vi "Outgoing Signals.vi"(8 "error in (no error)":errorcluster, 11 "Node Ptr":T4 format="%.0x") -> (0 "error out":errorcluster)   [LabVIEW 2009, in "NI-XNET Custom Device.lvlib"]
uses:
  NI-XNET Custom Device.lvlib
  <vilib>/NI VeriStand/Custom Device API/Custom Device Item Ref.ctl
  Add Selected.ctl
  Add All.ctl
  Browse for Channel.ctl
  <vilib>/xnet/xnet.llb/XNET String To IO Name (Frame).vi
  <vilib>/NI VeriStand/Custom Device API/Get Item Property (String).vi
  <vilib>/NI VeriStand/Custom Device API/Get Item Property (Boolean).vi
  <vilib>/NI VeriStand/Custom Device API/Custom Device Channel.ctl
  <vilib>/NI VeriStand/Custom Device API/Custom Device Channel Type.ctl
  <vilib>/NI VeriStand/Custom Device API/Set Item Property (Variant).vi
  <vilib>/NI VeriStand/Custom Device API/Set Item Property (Boolean).vi
  <vilib>/NI VeriStand/Custom Device API/Set Item Property (String).vi
  <vilib>/NI VeriStand/Custom Device API/Custom Device API.lvlib
  Program Files/National Instruments/LabVIEW 2009/resource/objmgr/xnet.rc
panel:
  in  "Enable Bool":bool
  in  "Header 6":cluster{"Section Name 2":string}={"Section Name 2"="Frame Timing"}
  out "Enable/Disable Channel":string
  in  "Add Enable":T1
  in  "Header 5":cluster{"Section Name":string}={"Section Name"="Signal Specifications"}
  in  "Header 4":cluster{"Section Name":string}={"Section Name"="Signal Values"}
  in  "Header 3":cluster{"Section Name":string}={"Section Name"="Signal Settings"}
  in  "Add All":T2
  in  "Add Signal":T3
  out "Unit":string
  out "Start Bit":u32
  out "Scaling Offset":dbl
  out "Scaling Factor":dbl
  out "Number of Bits":u32
  out "Minimum Value":dbl
  out "Maximum Value":dbl
  out "Default Value":dbl
  out "Data Type":u32(ring) items=["Signed", "Unsigned", "IEEE Float"]
  out "Comment":string
  out "Byte Order":u32(ring) items=["Little Endian", "Big Endian"]
  in  "Signal Selection":i32(listbox)
  in  "Header":cluster{"Section Name":string}={"Section Name"="Signal Selection"}
  in  "Delete":bool
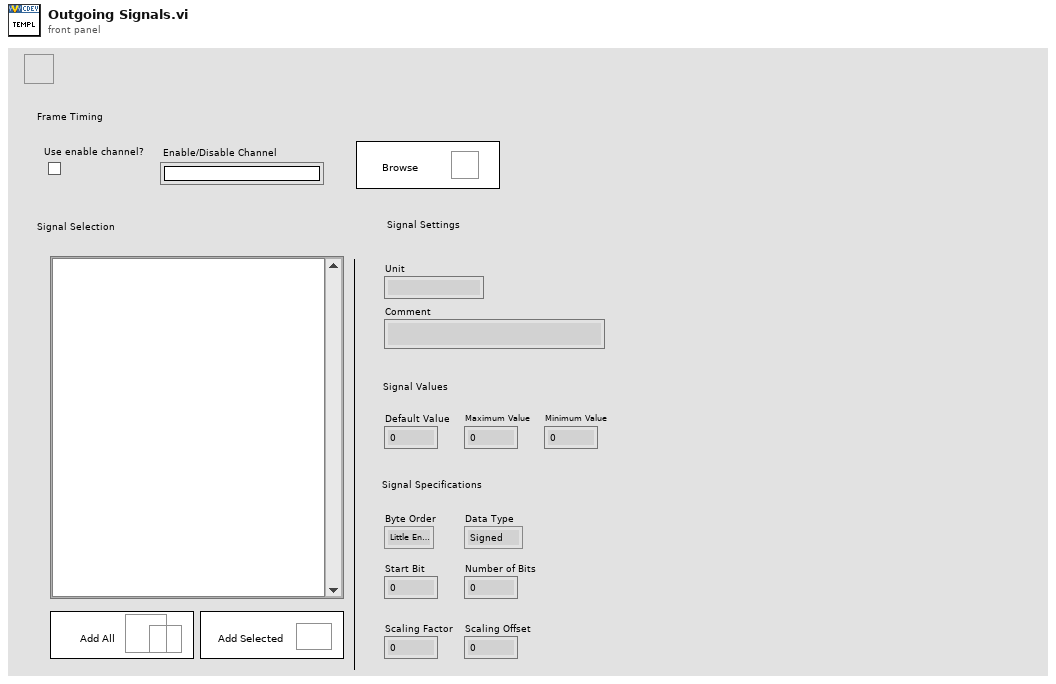
[diagram p1: front panel]
types:
  T1 = typedef "NI-XNET Custom Device.lvlib/Browse for Channel.ctl" = bool
  T2 = typedef "NI-XNET Custom Device.lvlib/Add All.ctl" = bool
  T3 = typedef "NI-XNET Custom Device.lvlib/Add Selected.ctl" = bool
  T4 = typedef "Custom Device API.lvlib/Custom Device Item Ref.ctl" = u64
  T5 = typedef "Custom Device API.lvlib/Custom Device Channel.ctl" = cluster{"Type":T6, "Units":string, "Default Value":dbl, "Faultable":bool, "Scalable":bool}
  T6 = typedef "Custom Device API.lvlib/Custom Device Channel Type.ctl" = enum16{"Input", "Output"}
  T7 = typedef "Custom Device API.lvlib/Custom Device Commands.ctl" = enum16{"Default", "Item renamed", "Shutdown"}
  T8 = typedef "Custom Device API.lvlib/Custom Device Item Info.ctl" = cluster{"Name":string, "Is Channel":bool, "GUID":string}
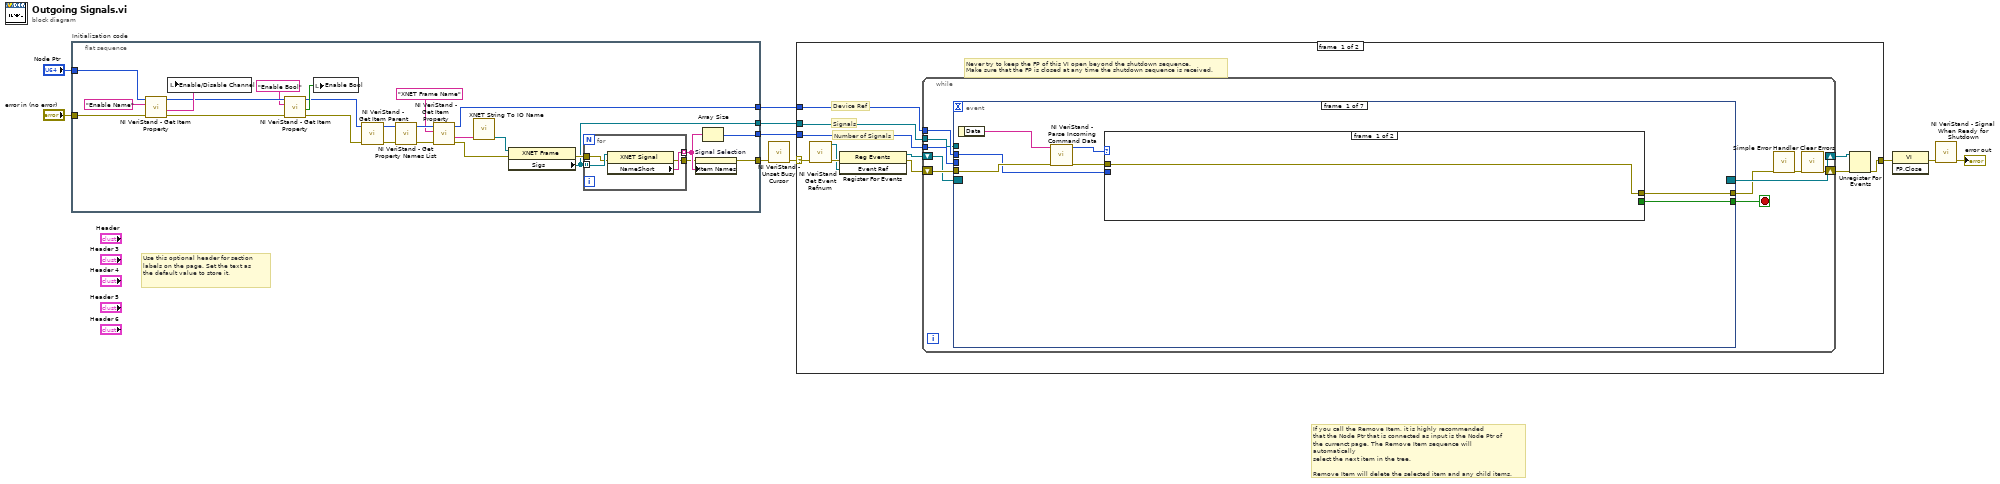
[diagram p0: block diagram]
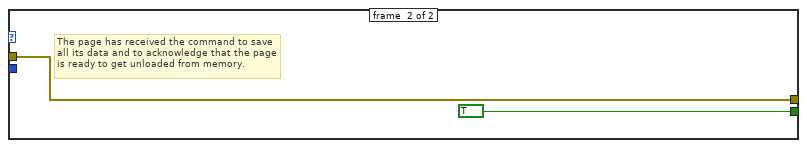
[diagram p2: hidden frame]
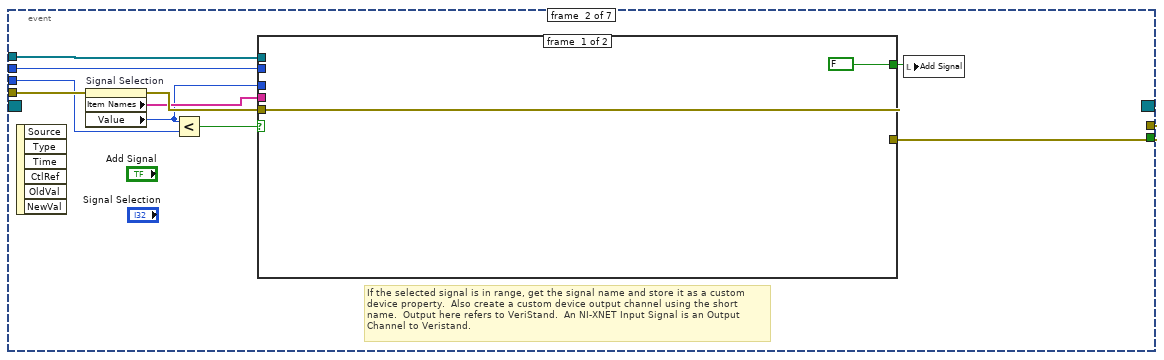
[diagram p3: hidden frame]
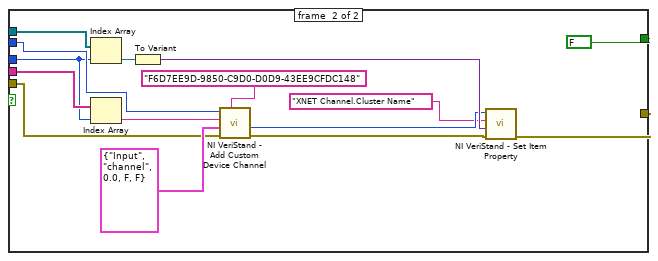
[diagram p4: hidden frame]
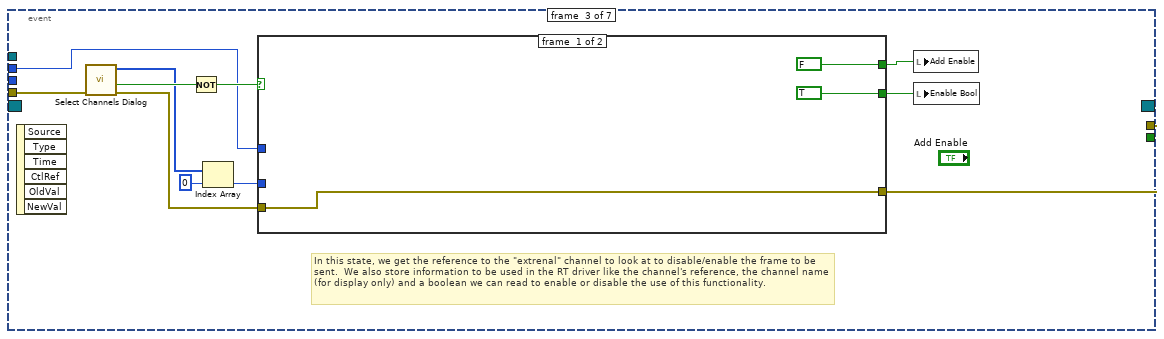
[diagram p5: hidden frame]
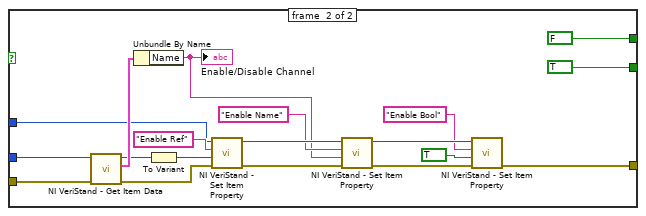
[diagram p6: hidden frame]
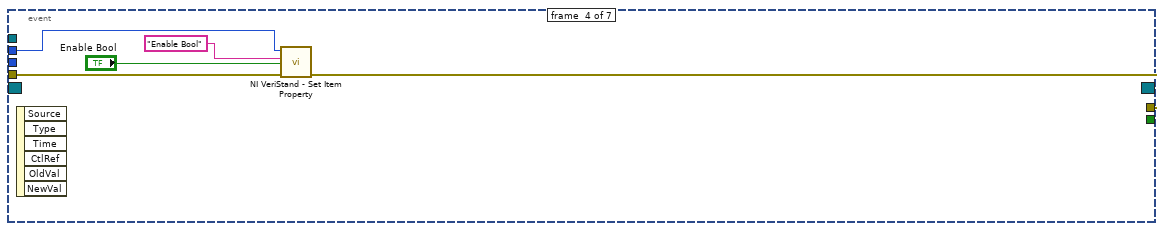
[diagram p7: hidden frame]
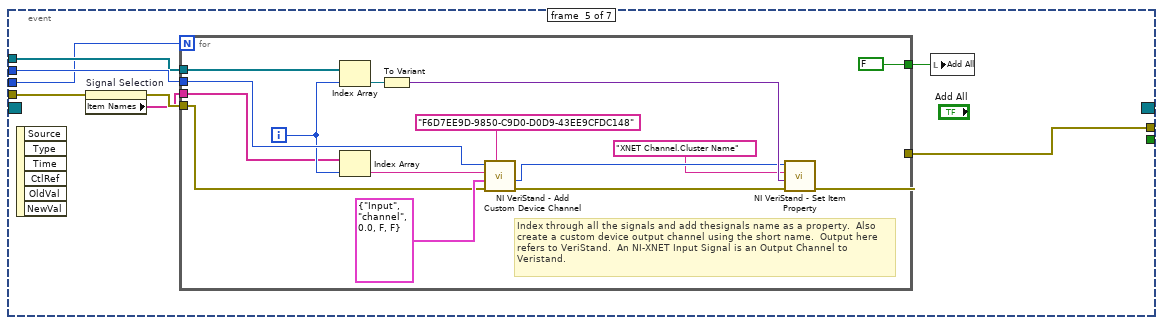
[diagram p8: hidden frame]
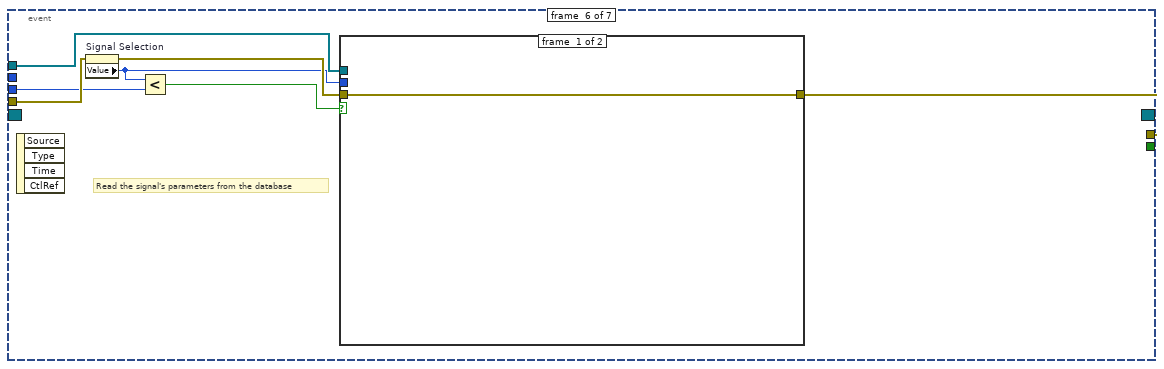
[diagram p9: hidden frame]
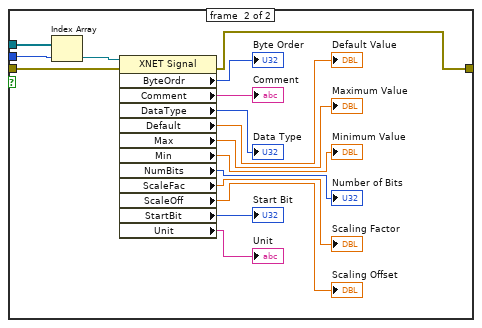
[diagram p10: hidden frame]
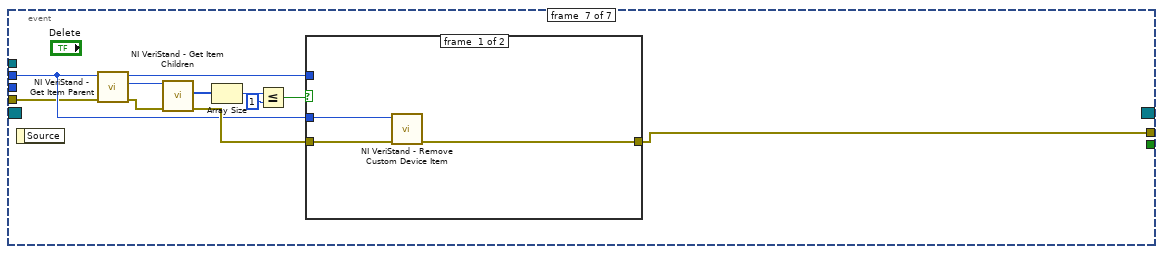
[diagram p11: hidden frame]
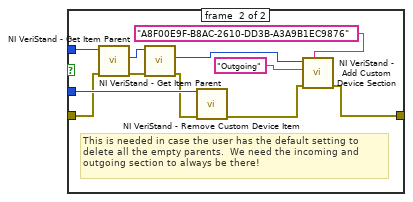
[diagram p12: hidden frame]
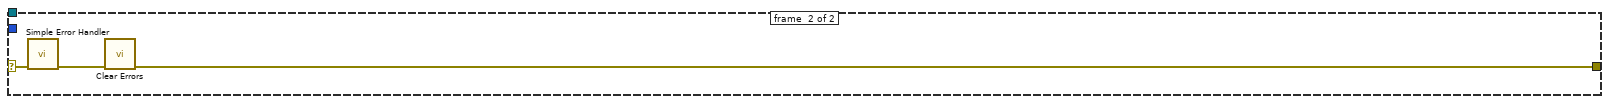
[diagram p13: hidden frame]
diagram:
  # "If you call the Remove Item, it is highly recommended\nthat the Node Ptr that is connected as input is the Node Ptr of\nthe currenct page. The Remove Item sequence will automatically\nselect the next item in the tree.\n\nRemove Item will delete the selected item and any child items."
  # "Use this optional header for section labels on the page. Set the text as the default value to store it."
  n1 = flat-sequence "Initialization code" {
    tunnel: "error in (no error)" -> [w25]
    tunnel: "Node Ptr" -> [w22]
    tunnel: [w13] -> w6
    tunnel: [w11] -> w3
    tunnel: [w27] -> w1
    tunnel: [w26] -> w2
    frame #0 {
      n2 = call-poly <vilib>:"NI VeriStand - Get Item Property.vi"("error in (no error)"=w25, "Property Name"="Enable Name", "Item Ref in"=w22) -> ("error out"=w20:errorcluster, "Value"=w24:string, "Item Ref out"=w21:T4)  [unwired: 5 in, 1 out]
      n3 = local write "Enable/Disable Channel"(w24) -> ()
      n4 = call-poly <vilib>:"NI VeriStand - Get Item Property.vi"("error in (no error)"=w20, "Property Name"="Enable Bool", "Item Ref in"=w21) -> ("error out"=w16:errorcluster, "Value"=w18:bool, "Item Ref out"=w17:T4)  [unwired: 5 in, 1 out]
      n5 = local write "Enable Bool"(w18) -> ()
      n6 = call <vilib>:"NI VeriStand - Get Item Parent.vi"("error in (no error)"=w16, "Parent Ref in"=w17) -> ("error out"=w29:errorcluster, "Parent Ref out"=w12:T4)  [unwired: 6 in, 2 out]
      n7 = call <vilib>:"NI VeriStand - Get Property Names List.vi"("error in (no error)"=w29, "Item Ref in"=w12) -> ("error out"=w31:errorcluster, "Item Ref out"=w30:T4)  [unwired: 7 in, 1 out]
      n8 = call-poly <vilib>:"NI VeriStand - Get Item Property.vi"("error in (no error)"=w31, "Property Name"="XNET Frame Name", "Item Ref in"=w30) -> ("error out"=w33:errorcluster, "Value"=w35:string, "Item Ref out"=w11:T4)  [unwired: 5 in, 1 out]
      n9 = call-poly <vilib>:"XNET String To IO Name.vi"("string"=w35) -> ("XNET Frame"=w32:refnum<k21>)  [unwired: 4 in]
      n10 = property class="XNET Frame"(reference=w32, error in=w33) -> (error out=w34:errorcluster, "Sigs"=w27:refnum<k21>[])  [unwired: 1 out]
      n11 = for {
        tunnel: w27 -> [w39] mode=indexing
        tunnel: [w38] -> w15 mode=indexing
        tunnel: w34 -> [w37]
        tunnel: [w36] -> w14
        n12 = property class="XNET Signal"(reference=w39, error in=w37) -> (error out=w36:errorcluster, "NameShort"=w38:string)  [unwired: 1 out]
      }
      n13 = property on="Signal Selection" class="LstBox (strict)"(error in=w14, "Item Names"=w15) -> (error out=w13:errorcluster)  [unwired: 1 in, 1 out]
      n14 = Array Size(array=w15) -> (size(s)=w26:i32)
    }
  }
  n15 = call <vilib>:"NI VeriStand - Unset Busy Cursor.vi"("error in (no error)"=w6) -> ("error out"=w5:errorcluster)  [unwired: 10 out]
  n16 = case shown="No Error" w5 {
    selector: w5 -> [w43 w210]
    tunnel: [w47 w208] -> w10
    tunnel: w3 -> [w41 _]
    tunnel: w2 -> [w42 _]
    tunnel: w1 -> [w40 _]
    frame #0 {
      # "Number of Signals"
      # "Signals"
      # "Device Ref"
      # "Never try to keep the FP of this VI open beyond the shutdown sequence.\nMake sure that the FP is closed at any time the shutdown sequence is received."
      n17 = call <vilib>:"NI VeriStand - Get Event Refnum.vi"("error in (no error)"=w43) -> ("error out"=w50:errorcluster, "Event Ref"=w46:refnum<user-event>)  [unwired: 9 out]
      n18 = register-events(error in=w50, w46) -> (reference out=w44:refnum<event-registration>, error out=w45:errorcluster)  [unwired: 1 in]
      n19 = while {
        shift-right: [w54] -> w48
        shift-left: w45 -> [w59]
        shift-right: [w60] -> w49
        shift-left: w44 -> [w58]
        tunnel: w42 -> [w53]
        tunnel: w41 -> [w52]
        tunnel: w40 -> [w51]
        stop <- w57 stop-if-true
        n20 = event shown="[6] \"Delete\": Value Change" {
          selector: w58 -> [_ _ _ _ _ _ _]
          dyn-events: [_ _ _ _ _ _ _] -> w60
          timeout: _ -> [_ _ _ _ _ _ _]
          tunnel: w59 -> [w67 w80 w102 w134 w138 w165 w184]
          tunnel: [w63 _ _ _ _ _ _] -> w57
          tunnel: [w62 w74 w100 w132 w141 w160 w183] -> w56
          tunnel: w53 -> [_ w73 _ _ w140 w164 _]
          tunnel: w52 -> [w61 w77 w101 w131 w143 _ w185]
          tunnel: w51 -> [_ w76 _ _ w142 w161 _]
          event #0 {
            n21 = event-data() -> ("Data"=w66:string)  [unwired: 1 out]
            n22 = call <vilib>:"NI VeriStand - Parse Incoming Command Data.vi"("error in (no error)"=w67, "Data"=w66) -> ("error out"=w65:errorcluster, "Action"=w64:T7)  [unwired: 8 out]
            n23 = case shown="\"Shutdown\"" w64 {
              tunnel: w65 -> [w68 w69]
              tunnel: [_ TRUE] -> w63
              tunnel: [w68 w69] -> w62
              tunnel: w61 -> [_ _]
              frame #0 {
              }
              frame #1 {
                # "The page has received the command to save all its data and to acknowledge that the page is ready to get unloaded from memory."
              }
            }
          }
          event #1 {
            # "If the selected signal is in range, get the signal name and store it as a custom device property.  Also create a custom device output channel using the short name.  Output here refers to VeriStand.  An NI-XNET Input Signal is an Output Channel to Veristand."
            n24 = event-data() -> ()  [unwired: 7 out]
            n25 = property on="Signal Selection" class="LstBox (strict)"(error in=w80) -> (error out=w79:errorcluster, "Item Names"=w72:string[], "Value"=w71:i32)  [unwired: 1 in, 1 out]
            n26 = Less?(x=w71, y=w73) -> (x < y?=w78:bool)
            n27 = case shown="True" w78 {
              tunnel: w79 -> [w81 w90]
              tunnel: w77 -> [_ w89]
              tunnel: w76 -> [_ w88]
              tunnel: [FALSE ("Add Signal") FALSE ("Add Signal")] -> w75
              tunnel: [w81 w86] -> w74
              tunnel: w72 -> [_ w85]
              tunnel: w71 -> [_ w84]
              frame #0 {
              }
              frame #1 {
                n28 = Index Array(array=w88, index=w84) -> (element=w95:refnum<k21>)
                n29 = Index Array(array=w85, index=w84) -> (element=w83:string)
                n30 = To Variant(anything=w95) -> (Variant=w96:variant)
                n31 = call <vilib>:"NI VeriStand - Add Custom Device Channel.vi"("GUID (Default Channel)"="F6D7EE9D-9850-C9D0-D0D9-43EE9CFDC148", "error in (no error)"=w90, "Channel"=T5 {"Type"=enum."Input", "Units"="channel", "Default Value"=0.0, "Faultable"=FALSE, "Scalable"=FALSE}, "Channel Name"=w83, "Parent Ref in"=w89) -> ("error out"=w97:errorcluster, "Channel Ref"=w94:T4)  [unwired: 4 in, 1 out]
                n32 = call-poly <vilib>:"NI VeriStand - Set Item Property.vi"("error in (no error)"=w97, "Value"=w96, "Property Name"="XNET Channel.Cluster Name", "Item Ref in"=w94) -> ("error out"=w86:errorcluster)  [unwired: 5 in, 2 out]
              }
            }
            n33 = local write "Add Signal"(w75) -> ()
          }
          event #2 {
            # "In this state, we get the reference to the \"extrenal\" channel to look at to disable/enable the frame to be sent.  We also store information to be used in the RT driver like the channel's reference, the channel name (for display only) and a boolean we can read to enable or disable the use of this functionality."
            n34 = event-data() -> ()  [unwired: 7 out]
            n35 = call "Select Channels Dialog.vi"("error in (no error)"=w102) -> ("error out"=w108:errorcluster, "Canceled"=w106:bool, "Selected Channel Refs"=w103:T4[])  [unwired: 8 in]
            n36 = Not(x=w106) -> (.not. x?=w107:bool)
            n37 = Index Array(array=w103, index=0) -> (element=w105:T4)
            n38 = case shown="True" w107 {
              tunnel: w105 -> [_ w130]
              tunnel: w108 -> [w111 w129]
              tunnel: w101 -> [_ w112]
              tunnel: [w111 w122] -> w100
              tunnel: [FALSE ("Add Enable") FALSE ("Add Enable")] -> w99
              tunnel: [TRUE ("Add Enable") TRUE ("Add Enable")] -> w98
              frame #0 {
              }
              frame #1 {
                n39 = call <vilib>:"NI VeriStand - Get Item Data.vi"("error in (no error)"=w129, "Item Ref in"=w130) -> ("error out"=w127:errorcluster, "Item Info"=w128:T8, "Item Ref out"=w114:T4)  [unwired: 7 out]
                n40 = Unbundle By Name(w128) -> ("Name"=w115:string)
                "Enable/Disable Channel" <- w115
                n41 = To Variant(anything=w114) -> (Variant=w113:variant)
                n42 = call-poly <vilib>:"NI VeriStand - Set Item Property.vi"("error in (no error)"=w127, "Value"=w113, "Property Name"="Enable Ref", "Item Ref in"=w112) -> ("error out"=w124:errorcluster, "Item Ref out"=w125:T4)  [unwired: 6 out]
                n43 = call-poly <vilib>:"NI VeriStand - Set Item Property.vi"("error in (no error)"=w124, "Value"=w115, "Property Name"="Enable Name", "Item Ref in"=w125) -> ("error out"=w121:errorcluster, "Item Ref out"=w120:T4)  [unwired: 6 out]
                n44 = call-poly <vilib>:"NI VeriStand - Set Item Property.vi"("error in (no error)"=w121, "Value"=TRUE, "Property Name"="Enable Bool", "Item Ref in"=w120) -> ("error out"=w122:errorcluster)  [unwired: 7 out]
              }
            }
            n45 = local write "Add Enable"(w99) -> ()
            n46 = local write "Enable Bool"(w98) -> ()
          }
          event #3 {
            n47 = event-data() -> ()  [unwired: 7 out]
            n48 = call-poly <vilib>:"NI VeriStand - Set Item Property.vi"("error in (no error)"=w134, "Value"="Enable Bool", "Property Name"="Enable Bool", "Item Ref in"=w131) -> ("error out"=w132:errorcluster)  [unwired: 7 out]
          }
          event #4 {
            n49 = event-data() -> ()  [unwired: 7 out]
            n50 = property on="Signal Selection" class="LstBox (strict)"(error in=w138) -> (error out=w137:errorcluster, "Item Names"=w136:string[])  [unwired: 1 in, 1 out]
            n51 = for {
              N: w140 -> [_]
              tunnel: w143 -> [w158]
              tunnel: w142 -> [w157]
              tunnel: [FALSE ("Add Signal")] -> w139
              tunnel: w137 -> [w145]
              tunnel: [w148] -> w141
              tunnel: w136 -> [w146]
              i -> [w147]
              # "Index through all the signals and add thesignals name as a property.  Also create a custom device output channel using the short name.  Output here refers to VeriStand.  An NI-XNET Input Signal is an Output Channel to Veristand."
              n52 = Index Array(array=w157, index=w147) -> (element=w153:refnum<k21>)
              n53 = Index Array(array=w146, index=w147) -> (element=w144:string)
              n54 = To Variant(anything=w153) -> (Variant=w154:variant)
              n55 = call <vilib>:"NI VeriStand - Add Custom Device Channel.vi"("GUID (Default Channel)"="F6D7EE9D-9850-C9D0-D0D9-43EE9CFDC148", "error in (no error)"=w145, "Channel"=T5 {"Type"=enum."Input", "Units"="channel", "Default Value"=0.0, "Faultable"=FALSE, "Scalable"=FALSE}, "Channel Name"=w144, "Parent Ref in"=w158) -> ("error out"=w155:errorcluster, "Channel Ref"=w152:T4)  [unwired: 4 in, 1 out]
              n56 = call-poly <vilib>:"NI VeriStand - Set Item Property.vi"("error in (no error)"=w155, "Value"=w154, "Property Name"="XNET Channel.Cluster Name", "Item Ref in"=w152) -> ("error out"=w148:errorcluster)  [unwired: 5 in, 2 out]
            }
            n57 = local write "Add All"(w139) -> ()
          }
          event #5 {
            # "Read the signal's parameters from the database"
            n58 = event-data() -> ()  [unwired: 5 out]
            n59 = property on="Signal Selection" class="LstBox (strict)"(error in=w165) -> (error out=w162:errorcluster, "Value"=w159:i32)  [unwired: 1 in, 1 out]
            n60 = Less?(x=w159, y=w164) -> (x < y?=w163:bool)
            n61 = case shown="True" w163 {
              tunnel: w162 -> [w166 w182]
              tunnel: w161 -> [_ w181]
              tunnel: [w166 w169] -> w160
              tunnel: w159 -> [_ w167]
              frame #0 {
              }
              frame #1 {
                n62 = Index Array(array=w181, index=w167) -> (element=w180:refnum<k21>)
                n63 = property class="XNET Signal"(reference=w180, error in=w182) -> (error out=w169:errorcluster, "ByteOrdr"=→"Byte Order":u32, "Comment"=→"Comment":string, "DataType"=→"Data Type":u32, "Default"=→"Default Value":dbl, "Max"=→"Maximum Value":dbl, "Min"=→"Minimum Value":dbl, "NumBits"=→"Number of Bits":u32, "ScaleFac"=→"Scaling Factor":dbl, "ScaleOff"=→"Scaling Offset":dbl, "StartBit"=→"Start Bit":u32, "Unit"=→"Unit":string)  [unwired: 1 out]
              }
            }
          }
          event #6 {
            n64 = event-data() -> ()  [unwired: 2 out]
            n65 = call <vilib>:"NI VeriStand - Get Item Parent.vi"("error in (no error)"=w184, "Parent Ref in"=w185) -> ("error out"=w187:errorcluster, "Parent Ref"=w186:T4, "Parent Ref out"=w193:T4)  [unwired: 6 in, 1 out]
            n66 = call <vilib>:"NI VeriStand - Get Item Children.vi"("error in (no error)"=w187, "Item Ref in"=w186) -> ("error out"=w191:errorcluster, "Child Refs"=w188:T4[])  [unwired: 6 in, 2 out]
            n67 = Array Size(array=w188) -> (size(s)=w189:i32)
            n68 = Less Or Equal?(x=w189, y=1) -> (x <= y?=w192:bool)
            n69 = case shown="True" w192 {
              tunnel: [w196 w204] -> w183
              tunnel: w185 -> [w195 w206]
              tunnel: w191 -> [w194 w201]
              tunnel: w193 -> [_ w207]
              frame #0 {
                n70 = call <vilib>:"NI VeriStand - Remove Custom Device Item.vi"("error in (no error)"=w194, "Item Ref in"=w195) -> ("error out"=w196:errorcluster)  [unwired: 1 in, 8 out]
              }
              frame #1 {
                # "This is needed in case the user has the default setting to delete all the empty parents.  We need the incoming and outgoing section to always be there!"
                n71 = call <vilib>:"NI VeriStand - Get Item Parent.vi"("error in (no error)"=w201, "Parent Ref in"=w207) -> ("error out"=w200:errorcluster, "Parent Ref"=w198:T4)  [unwired: 6 in, 2 out]
                n72 = call <vilib>:"NI VeriStand - Get Item Parent.vi"("error in (no error)"=w200, "Parent Ref in"=w198) -> ("error out"=w199:errorcluster, "Parent Ref"=w197:T4)  [unwired: 6 in, 2 out]
                n73 = call <vilib>:"NI VeriStand - Remove Custom Device Item.vi"("error in (no error)"=w199, "Item Ref in"=w206) -> ("error out"=w205:errorcluster)  [unwired: 1 in, 8 out]
                n74 = call <vilib>:"NI VeriStand - Add Custom Device Section.vi"("GUID (Default Section)"="A8F00E9F-B8AC-2610-DD3B-A3A9B1EC9876", "error in (no error)"=w205, "Section Name"="Outgoing", "Parent Ref in"=w197) -> ("error out"=w204:errorcluster)  [unwired: 5 in, 2 out]
              }
            }
          }
        }
        n75 = call <vilib>:"Simple Error Handler.vi"("error in (no error)"=w56) -> ("error out"=w55:errorcluster)  [unwired: 1 in, 7 out]
        n76 = call <vilib>:"Clear Errors.vi"("error in (no error)"=w55) -> ("error out"=w54:errorcluster)  [unwired: 6 out]
      }
      n77 = Unregister For Events(event registration refnum=w49, error in=w48) -> (error out=w47:errorcluster)
    }
    frame #1 {
      n78 = call <vilib>:"Simple Error Handler.vi"("error in (no error)"=w210) -> ("error out"=w209:errorcluster)  [unwired: 1 in, 7 out]
      n79 = call <vilib>:"Clear Errors.vi"("error in (no error)"=w209) -> ("error out"=w208:errorcluster)  [unwired: 6 out]
    }
  }
  n80 = invoke class="VI" method="FP.Close"(error in=w10) -> (error out=w9:errorcluster)  [unwired: 2 in, 2 out]
  n81 = call <vilib>:"NI VeriStand - Signal When Ready for Shutdown.vi"("error in (no error)"=w9) -> ("error out"=→"error out":errorcluster)  [unwired: 10 out]
